vi "Run_Init Core.vi"(0 "Structure Loop in":refnum<class "Structure Loop.lvclass">, 11 "error in (no error)":errorcluster) -> (4 "Structure Loop out":refnum<class "Structure Loop.lvclass">, 15 "error out":errorcluster)   [LabVIEW 2016, in "Structure Loop.lvclass"]
uses:
  Structure Loop.lvclass
  E:/Repository/LabVIEW Script Language/source code/LSL components/functions/functionsbase/functionbase.lvclass
  Structure Loop.lvclass/Structure Loop.ctl
  functionsbase/functionbase.lvclass
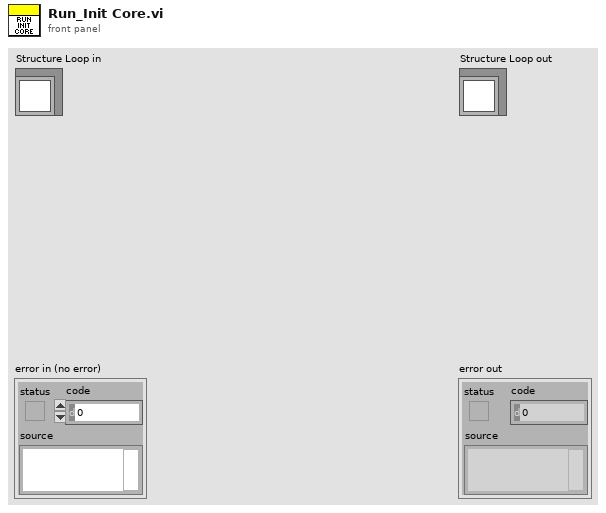
[diagram p1: front panel]
types:
  T1 = typedef "Valuetype.ctl" = enum16{"Value", "Variable", "Function"}
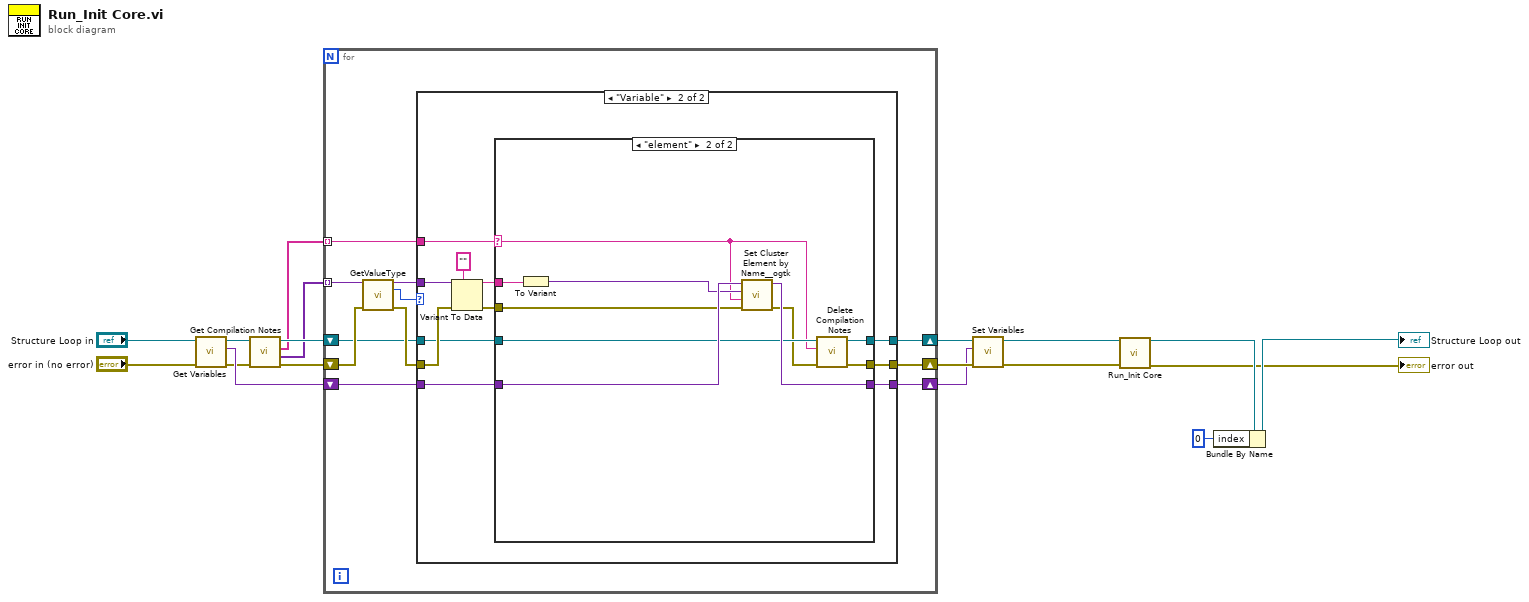
[diagram p0: block diagram]
diagram:
  n1 = call-dynamic "Get Variables.vi"("error in (no error)"="error in (no error)", "For Loop in"="Structure Loop in") -> ("error out"=w12:errorcluster, "Variables"=w16:variant, "For Loop out"=w11:refnum<class "Structure Loop.lvclass">)  [unwired: 7 in]
  n2 = call "Get Compilation Notes.vi"("error in (no error)"=w12, "functionbase in"=w11) -> ("error out"=w10:errorcluster, "note"=w8:variant[], "note Key"=w7:string[], "functionbase out"=w9:refnum<class "Structure Loop.lvclass">)  [unwired: 6 in]
  n3 = for {
    shift-right: [w19] -> w15
    shift-left: w9 -> [w20]
    shift-right: [w28] -> w13
    shift-left: w16 -> [w29]
    shift-right: [w27] -> w14
    shift-left: w10 -> [w25]
    tunnel: w8 -> [w26] mode=indexing
    tunnel: w7 -> [w24] mode=indexing
    n4 = call "GetValueType.vi"("variant"=w26, "error in"=w25) -> ("variant out"=w22:variant, "Value Type"=w23:T1, "error out"=w21:errorcluster)  [unwired: 11 in]
    n5 = case shown="\"Variable\"" w23 {
      tunnel: w22 -> [_ w42]
      tunnel: [w32 w37] -> w28
      tunnel: w29 -> [w32 w38]
      tunnel: [w31 w36] -> w27
      tunnel: w21 -> [w31 w43]
      tunnel: w24 -> [_ w35]
      tunnel: w20 -> [w30 w34]
      tunnel: [w30 w33] -> w19
      frame Default {
      }
      frame "Variable" {
        n6 = Variant To Data(error in=w43, type="", Variant=w42) -> (data=w39:string, error out=w40:errorcluster)
        n7 = case shown="\"element\"" w35 {
          selector: w35 -> [_ w47]
          tunnel: w40 -> [w45 w54]
          tunnel: w39 -> [_ w53]
          tunnel: w38 -> [w46 w56]
          tunnel: [w46 w55] -> w37
          tunnel: [w45 w48] -> w36
          tunnel: w34 -> [w44 w51]
          tunnel: [w44 w50] -> w33
          frame Default {
          }
          frame "element" {
            n8 = To Variant(anything=w53) -> (Variant=w52:variant)
            n9 = call <userlib>:"Set Cluster Element by Name__ogtk.vi"("error in (no error)"=w54, "Element Name (\"\": New Element Data Name)"=w47, "New Element Value"=w52, "Cluster"=w56) -> ("error out"=w49:errorcluster, "VCluster out"=w55:variant)  [unwired: 5 in, 1 out]
            n10 = call "Delete Compilation Notes.vi"("error in (no error)"=w49, "note key"=w47, "functionbase in"=w51) -> ("error out"=w48:errorcluster, "functionbase out"=w50:refnum<class "Structure Loop.lvclass">)  [unwired: 7 in]
          }
        }
      }
    }
  }
  n11 = call-dynamic "Set Variables.vi"("error in (no error)"=w14, "Variables"=w13, "For Loop in"=w15) -> ("error out"=w2:errorcluster, "For Loop out"=w4:refnum<class "Structure Loop.lvclass">)  [unwired: 7 in]
  n12 = call-parent "Run_Init Core.vi"("functionbase in"=w4, "error in (no error)"=w2) -> ("functionbase out"=w3:refnum<class "Structure Loop.lvclass">, "error out"=→"error out":errorcluster)  [unwired: 12 in]
  n13 = Bundle By Name(cluster=w3, "index"=0) -> (→"Structure Loop out":refnum<class "Structure Loop.lvclass">)
